vi "RSZVB Set User Connector.vi"(6 "Connector":string, 7 "Connector Gender (0: Male)":i32(ring)=1 items=["Male", "Female"], 8 "error in (no error)":errorcluster {"code" format="%.0x"}, 9 "Port (1)":i32=1, 10 "Channel (1)":i32=1, 11 "VISA session":refnum<visa-resource-name>) -> (0 "error out":errorcluster {"code" format="%.0x"}, 3 "dup VISA session":refnum<visa-resource-name>)   [LabVIEW 2011]
doc: "This VI selects a user-defined connector type at a specified port <Port> and its gender.\n\nRemote-control command(s):\n[SENSe<Ch>:]CORRection:COLLect:SCONnection<port_no> '<conn_name>', MALE | FEMale"
uses:
  _utility/RSZVB Global Data.vi
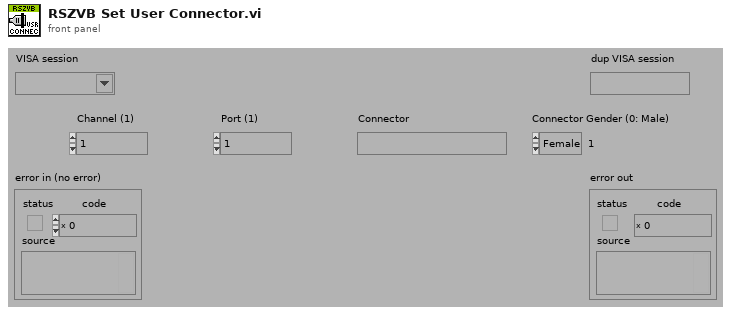
[diagram p1: front panel]
types:
  T1 = cluster{"Error Checking (T: On)":bool, "Installed Options":string[], "Data Valid?":bool, "Ports":i32, "Model":string[], "Option Checking (T: On)":bool}[]
  T2 = cluster{"Error Checking (T: On)":bool, "Installed Options":string[], "Data Valid?":bool, "Ports":i32, "Model":string[], "Option Checking (T: On)":bool}
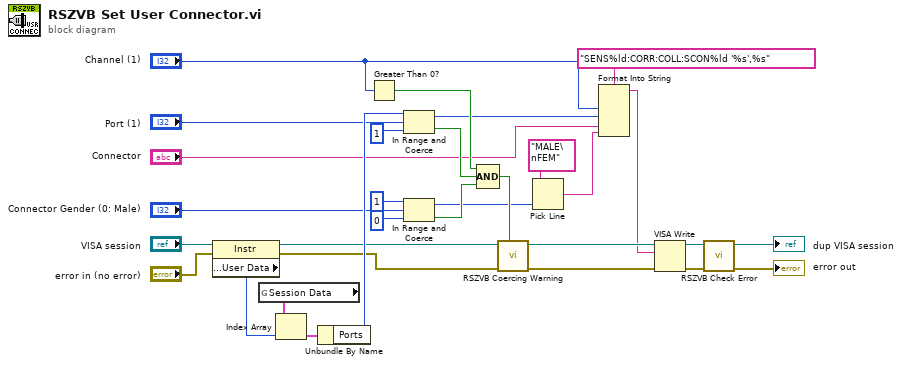
[diagram p0: block diagram]
diagram:
  n1 = property class="Instr"(reference="VISA session", error in="error in (no error)") -> (reference out=w2:refnum<visa-resource-name>, error out=w1:errorcluster, "General Settings:User Data"=w19:u32)
  n2 = global read "RSZVB Global Data.vi" "Session Data"() -> (w20:T1)
  n3 = Index Array(array=w20, index=w19) -> (element=w21:T2)
  n4 = Unbundle By Name(w21) -> ("Ports"=w16:i32)
  n5 = Greater Than 0?(x="Channel (1)") -> (x > 0?=w22:bool)
  n6 = In Range and Coerce(upper limit=w16, x="Port (1)", lower limit=1) -> (coerced(x)=w14:i32, In Range?=w25:bool)
  n7 = In Range and Coerce(upper limit=1 ("lower limit"), x="Connector Gender (0: Male)", lower limit=0) -> (coerced(x)=w12:i32, In Range?=w17:bool)
  n8 = Compound Arithmetic op=AND(w22, w25, w17) -> (w24:bool)
  n9 = call "RSZVB Coercing Warning.vi"("In Range?"=w24, "error in (no error)"=w1, "VISA session"=w2) -> ("error out"=w28:errorcluster, "dup VISA session"=w29:refnum<visa-resource-name>)  [unwired: 7 in]
  n10 = Pick Line(multi-line string="MALE\nFEM", line index=w12) -> (output string=w11:string)  [unwired: 1 in]
  n11 = Format Into String(format string="SENS%ld:CORR:COLL:SCON%ld '%s',%s", "Channel (1)", w14, "Connector", w11) -> (resulting string=w23:string)  [unwired: 2 in, 1 out]
  n12 = VISA Write(VISA resource name=w29, write buffer=w23, error in (no error)=w28) -> (VISA resource name out=w26:refnum<visa-resource-name>, error out=w27:errorcluster)  [unwired: 1 out]
  n13 = call "RSZVB Check Error.vi"("error in (no error)"=w27, "VISA session"=w26) -> ("error out"=→"error out":errorcluster, "dup VISA session"=→"dup VISA session":refnum<visa-resource-name>)  [unwired: 8 in]
